vi "PH_Beckhoff.set Analog Intputs Defaults.vi"(1 "Service IDs":i32[](array[numeric]), 2 "Sca Type":u32[](array[numeric]), 3 "Analog Input Tag Names":string[](array[string])) -> (0 "Analog Inputs":T2)   [LabVIEW 2014, in "PH_Beckhoff.lvlib"]
uses:
  PH_Beckhoff.lvlib
  PH_Beckhoff.Analog Inputs.ctl
  PH_Beckhoff.Scaling Type.ctl
panel:
  in  "Analog Input Value":T1={"Name"="", "Value"=0, "Quality"=FALSE, "Service ID"=-1, "Sca Type"=0}
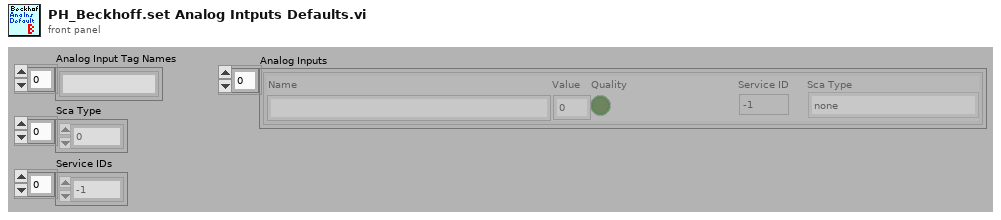
[diagram p1: front panel]
types:
  T1 = cluster{"Name":string, "Value":u32, "Quality":bool, "Service ID":i32, "Sca Type":u32}
  T2 = typedef "PH_Beckhoff.lvlib/PH_Beckhoff.Analog Inputs.ctl" = cluster{"Name":string, "Value":u32, "Quality":bool, "Service ID":i32, "Sca Type":T3}[]
  T3 = typedef "PH_Beckhoff.lvlib/PH_Beckhoff.Scaling Type.ctl" = enum16{"none", "0 ... 15 Bit -> 0 ... 5", "0 ... 15 Bit -> 0 ... 10", "0 ... 15 Bit -> 0 ... 25", "0 ... 15 Bit -> 4 ... 20", "0 ... 15 Bit -> 0 ... 1", "0 ... 15 Bit -> 0 ... 20000", "0 ... 15 Bit -> 0 ... 24000"}
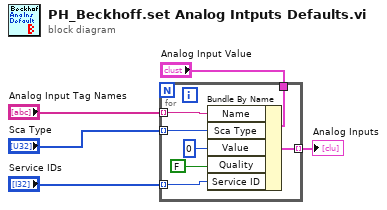
[diagram p0: block diagram]
diagram:
  n1 = for {
    tunnel: "Analog Input Value" -> [w12]
    tunnel: [w11] -> w2 mode=indexing
    tunnel: "Analog Input Tag Names" -> [w10] mode=indexing
    tunnel: "Sca Type" -> [w9] mode=indexing
    tunnel: "Service IDs" -> [w6] mode=indexing
    n2 = Bundle By Name(cluster=w12, "Name"=w10, "Sca Type"=w9, "Value"=u32 0, "Quality"=FALSE, "Service ID"=w6) -> (w11:T1)
  }
  "Analog Inputs" <- w2
